vi "Leaf.vi"(0 "Image In":T2, 7 "error in":errorcluster) -> (20 "Image Out":T2, 21 "Matches (Leaf)":T1(array[cluster]) {"Bounding Box"."y" format="%.2f"; "Bounding Box"."x" format="%.2f"; "Position"."y" format="%.2f"; "Position"."x" format="%.2f"; "Score" format="%.2f"; "Scale" format="%.2f"; "Angle" format="%.2f"}, 22 "Calibrated Matches (Leaf)":T1(array[cluster]) {"Bounding Box"."y" format="%.2f"; "Bounding Box"."x" format="%.2f"; "Position"."y" format="%.2f"; "Position"."x" format="%.2f"; "Score" format="%.2f"; "Scale" format="%.2f"; "Angle" format="%.2f"}, 23 "Number of Matches (Leaf)":i32, 27 "error out":errorcluster)   [LabVIEW 2012]
uses:
  <vilib>/vision/Image Controls.llb/IMAQ Image.ctl
  <vilib>/vision/NI_Vision_Development_Module.lvlib
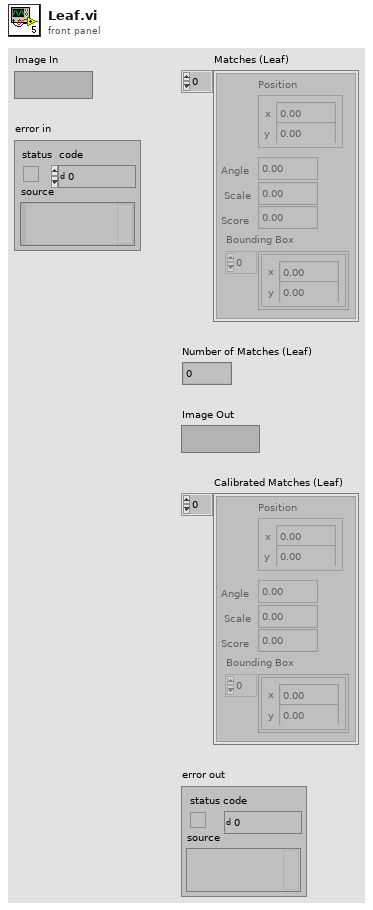
[diagram p1: front panel]
types:
  T1 = cluster{"Position":cluster{"x":sgl, "y":sgl}, "Angle":sgl, "Scale":sgl, "Score":sgl, "Bounding Box":cluster{"x":sgl, "y":sgl}[]}[]
  T2 = typedef "IMAQ Image.ctl" = refnum<image>
  T3 = typedef "Image Type" = u32
  T4 = cluster{"Global Rectangle":i32[], "Contours":cluster{"ID":enum32{"External", "Internal"}, "Type":u32, "Coordinates":i32[]}[]}
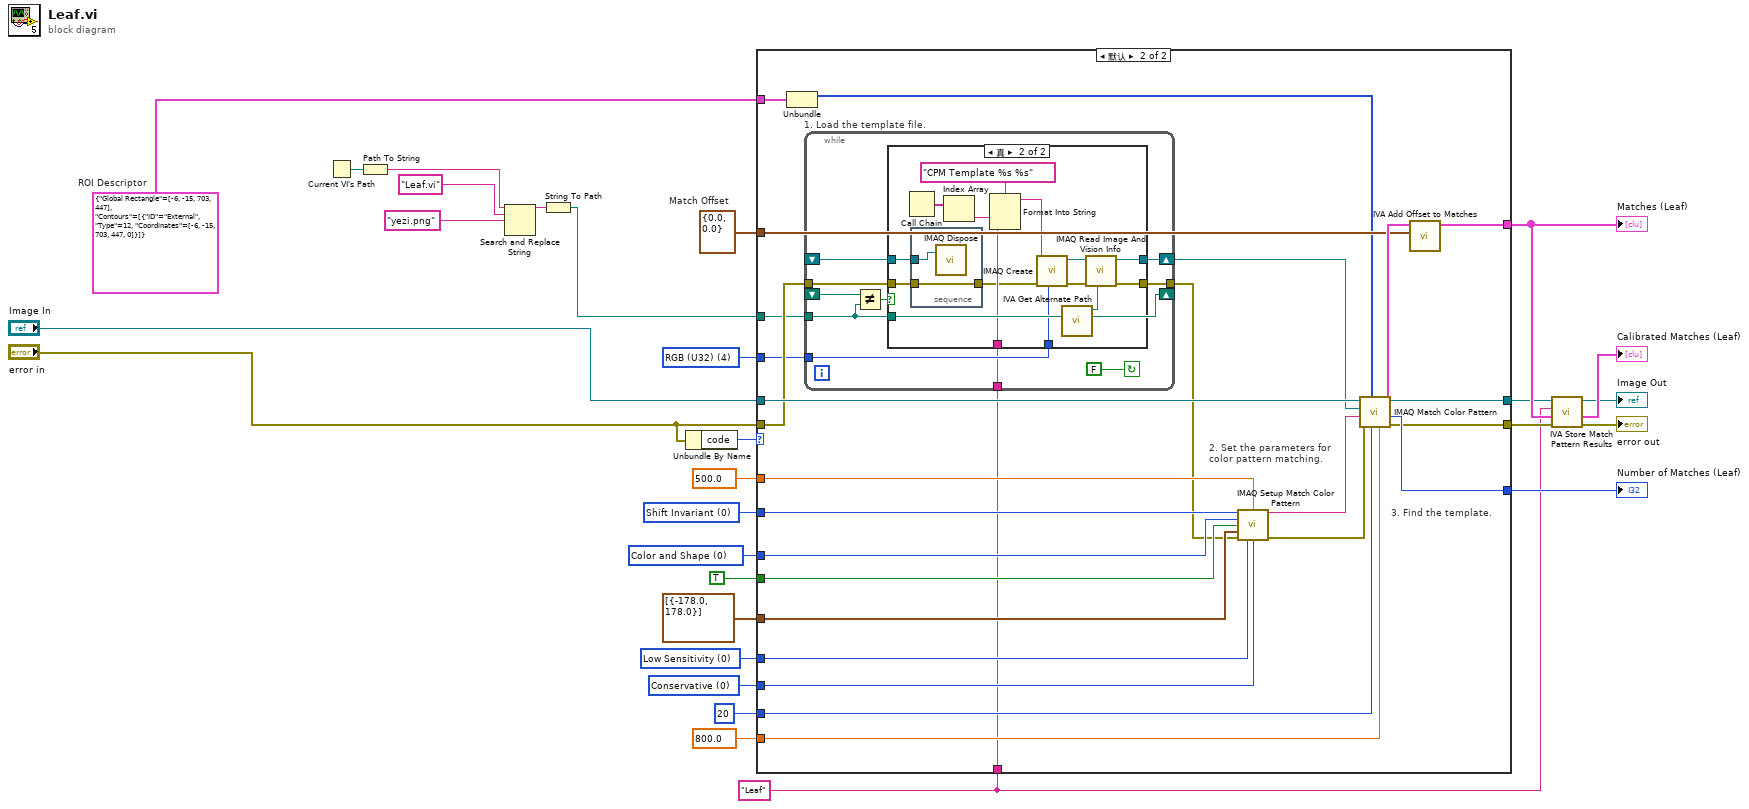
[diagram p0: block diagram]
diagram:
  w7 = "Leaf" ("Step Name")
  w19 = T3 4 items=["Grayscale (U8)", "Grayscale (I16)", "Grayscale (SGL)", "Complex (CSG)", "RGB (U32)", "HSL (U32)", "RGB (U64)"] ("Image Type")
  w17 = cluster{"X":sgl, "Y":sgl} {"X"=0.0, "Y"=0.0}  # Match Offset
  w21 = u32 0 items=["Conservative", "Balance", "Aggressive", "Very Aggressive"] ("Search Strategy")
  w22 = u32 0 items=["Low Sensitivity", "Medium Sensitivity", "High Sensitivity"] ("Color Sensitivity")
  w24 = u32 0 items=["Color and Shape", "Color", "Shape"] ("Match Feature Mode")
  w25 = u32 0 items=["Shift Invariant", "Rotation Invariant"] ("Match Mode")
  w16 = T4 {"Global Rectangle"=[-6, -15, 703, 447], "Contours"=[{"ID"=enum."External", "Type"=12, "Coordinates"=[-6, -15, 703, 447, 0]}]}  # ROI Descriptor
  n1 = Current VI's Path() -> (path=w6:path)
  n2 = Path To String(path=w6) -> (string=w5:string)
  n3 = Search and Replace String(input string=w5, search string="Leaf.vi", replace string="yezi.png") -> (result string=w2:string)  [unwired: 5 in, 3 out]
  n4 = String To Path(string=w2) -> (path=w1:path)
  n5 = Unbundle By Name("error in") -> ("code"=w14:i32)
  n6 = case "条件结构" shown="默认" w14 {
    tunnel: 20 ("Number of Matches Requested") -> [_ w55]
    tunnel: sgl 800.0 ("Minimum Match Score") -> [_ w54]
    tunnel: [_ w53] -> w26
    tunnel: w25 -> [_ w52]
    tunnel: w24 -> [_ w51]
    tunnel: TRUE ("Subpixel Accuracy") -> [_ w50]
    tunnel: w22 -> [_ w49]
    tunnel: w21 -> [_ w48]
    tunnel: sgl 500.0 ("Color Score Weight") -> [_ w47]
    tunnel: w1 -> [_ w36]
    tunnel: w19 -> [_ w32]
    tunnel: "error in" -> [_ w37]
    tunnel: cluster{sgl, sgl}[] [{-178.0, 178.0}] ("Rotation Angle Ranges (degrees)") -> [_ w44]
    tunnel: w17 -> [_ w42]
    tunnel: w16 -> [_ w41]
    tunnel: [_ w33] -> w11
    tunnel: "Image In" -> [w30 w38]
    tunnel: [w30 w38] -> w8
    tunnel: [_ w39] -> w13
    tunnel: w7 -> [_ w31]
    frame -1074396199, -1074396198 {
      # "Discard Coordinate System Error"
    }
    frame Default {
      # "2. Set the parameters for\ncolor pattern matching."
      # "3. Find the template."
      n7 = Unbundle(w41) -> ("Global Rectangle"=w40:i32[])  [unwired: 1 out]
      n8 = while "1. Load the template file." {
        shift-right: [w65] -> w35
        shift-left: _ -> [w64]
        tunnel: [w62] -> w34
        tunnel: w37 -> [w61]
        tunnel: w36 -> [w56]
        tunnel: w32 -> [w60]
        tunnel: w31 -> [w59]
        shift-right: [w56] -> _
        shift-left: _ -> [w58]
        stop <- FALSE continue-if-true
        n9 = Not Equal?(x=w58, y=w56) -> (x != y?=w57:bool)
        n10 = case "条件结构" shown="真" w57 {
          tunnel: [w67 w80] -> w65
          tunnel: w64 -> [w67 w72]
          tunnel: [w66 w77] -> w62
          tunnel: w61 -> [w66 w71]
          tunnel: w56 -> [_ w69]
          tunnel: w60 -> [_ w76]
          tunnel: w59 -> [_ w73]
          frame False {
          }
          frame True {
            n11 = Call Chain() -> (call chain=w75:string[])
            n12 = stacked-sequence "层叠式顺序结构" {
              tunnel: w72 -> [w84]
              tunnel: w71 -> [w83]
              tunnel: [w83] -> w70
              frame #0 {
                n13 = call "IMAQ Dispose"("Image"=w84) -> ()  [unwired: 2 in, 4 out]
              }
            }
            n14 = Index Array(array=w75) -> (element=w74:string)  [unwired: 1 in]
            n15 = Format Into String(format string="CPM Template %s %s" ("Image Name"), w74, w73) -> (resulting string=w82:string)  [unwired: 2 in, 1 out]
            n16 = call "IMAQ Create"("Image Name"=w82, "Image Type"=w76, "error in (no error)"=w70) -> ("New Image"=w79:T2, "error out"=w78:errorcluster)  [unwired: 1 in, 1 out]
            n17 = call <vilib>:"IVA Get Alternate Path.vi"("Path In"=w69) -> ("Path Out"=w68:path)  [unwired: 10 out]
            n18 = call "IMAQ Read Image And Vision Info"("File Path"=w68, "error in (no error)"=w78, "Image"=w79) -> ("error out"=w77:errorcluster, "Image Out"=w80:T2)  [unwired: 1 in, 6 out]
          }
        }
      }
      n19 = call "IMAQ Setup Match Color Pattern"("Match Mode"=w52, "Color Score Weight"=w47, "Match Feature Mode"=w51, "Subpixel Accuracy"=w50, "Rotation Angle Ranges (degrees)"=w44, "error in (no error)"=w34, "Color Sensitivity"=w49, "Search Strategy"=w48) -> ("Match Color Pattern Setup Data"=w46:string, "error out"=w45:errorcluster)  [unwired: 1 in, 5 out]
      n20 = call "IMAQ Match Color Pattern"("Minimum Match Score"=w54, "Number of Matches Requested"=w55, "Optional Rectangle"=w40, "error in (no error)"=w45, "Match Color Pattern Setup Data"=w46, "Template Image"=w35, "Image"=w38) -> ("error out"=w33:errorcluster, "Number of Matches"=w53:i32, "Matches"=w43:T1)  [unwired: 2 out]
      n21 = call <vilib>:"IVA Add Offset to Matches.vi"("Match Offset"=w42, "Matches in"=w43) -> ("Matches out"=w39:T1)  [unwired: 9 out]
    }
  }
  "Matches (Leaf)" <- w13
  "Number of Matches (Leaf)" <- w26
  n22 = call <vilib>:"IVA Store Match Pattern Results.vi"("error in (no error)"=w11, "Matches"=w13, "Step Name"=w7, "Image in"=w8) -> ("error out"=→"error out":errorcluster, "Calibrated Matches"=→"Calibrated Matches (Leaf)":T1, "Image dup"=→"Image Out":T2)  [unwired: 5 out]
